vi "pH电极校准.vi"() -> ()   [LabVIEW 2016, in "斯坦道多参数.lvlib"]
uses:
  <vilib>/Utility/miscctls.llb/LVPointTypeDef.ctl
  <vilib>/Analysis/NI_AALBase.lvlib
panel:
  in  "三点标液3":u16(ring)=6 caption="标液3" items=["TECH4.00", "TECH7.00", "TECH10.00", "NIST1.68", "NIST4.01", "NIST6.86", "NIST9.18", "NIST12.68"]
  in  "三点标液2":u16(ring)=5 caption="标液2" items=["TECH4.00", "TECH7.00", "TECH10.00", "NIST1.68", "NIST4.01", "NIST6.86", "NIST9.18", "NIST12.68"]
  in  "三点标液1":u16(ring)=4 caption="标液1" items=["TECH4.00", "TECH7.00", "TECH10.00", "NIST1.68", "NIST4.01", "NIST6.86", "NIST9.18", "NIST12.68"]
  out "第三点校准值":dbl
  in  "校准停止":bool
  in  "校准启动":bool
  out "第二点校准值":dbl
  out "第一点校准值":dbl
  out "提示":string
  in  "校准模式":enum16{"两点校准", "单点校准", "三点校准"}(ring)
  out "最小值":sgl format="%#.2f"
  out "最大值":sgl format="%#.2f"
  out "变异系数":dbl format="%#.6f"
  out "standard deviation":dbl caption="标准差" format="%#.2f"
  out "mean":dbl caption="均值" format="%#.2f"
  out "波形图表":sgl(graph) caption="历史曲线"
  out "当前检测值":dbl format="%#.2g"
  out "标液2":dbl
  out "标液1":dbl
  out "当前信号值":dbl format="%#.2g"
  out "偏移值补偿":dbl format="%#.2g"
  out "电极斜率":dbl
  out "电极零点":dbl
  # "酸碱度电极设定"
  # "mV"
  # "mV"
  # "%"
  # "pH"
  # "请选择校准模式:"
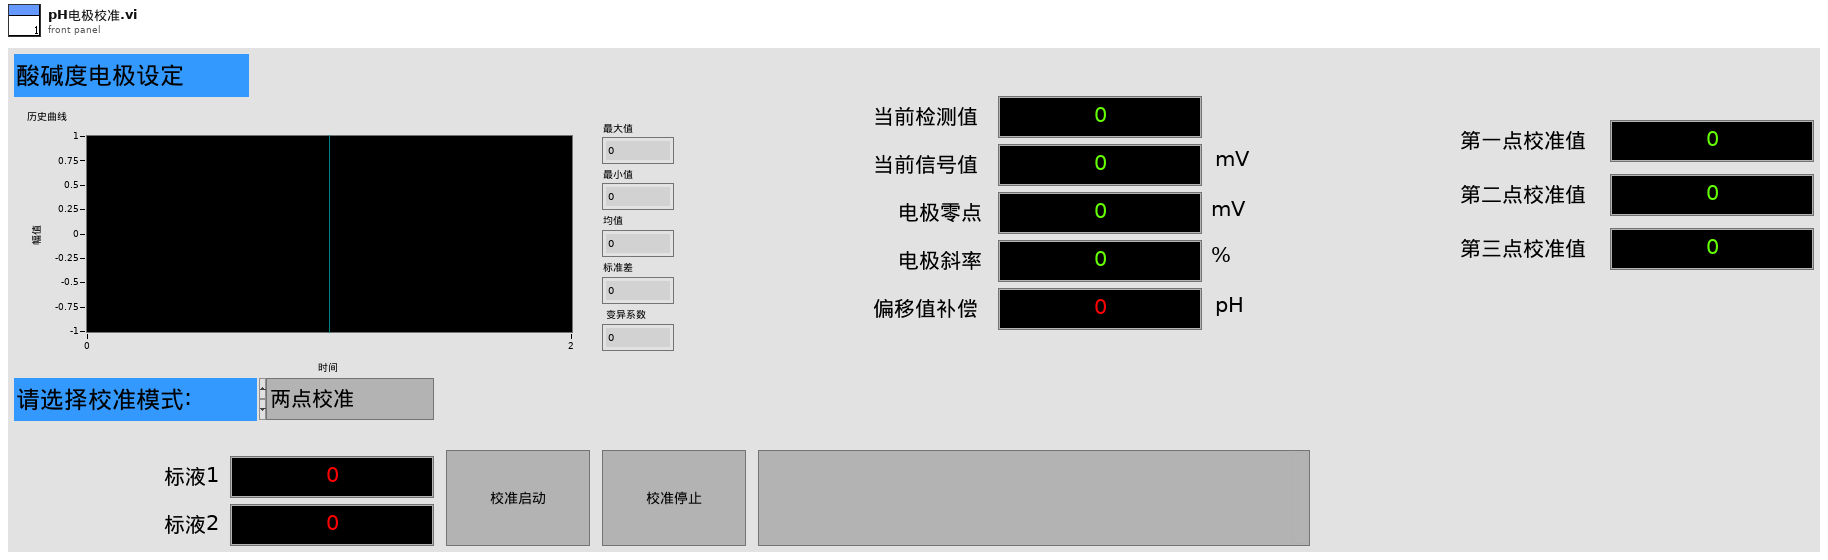
[diagram p1: front panel]
types:
  T1 = typedef "LVPointTypeDef.ctl" = cluster{"Horizontal":i16, "Vertical":i16}
  T2 = typedef "斯坦道多参数.lvlib/校准步骤.ctl" = enum16{"待机", "放置第一点标液", "第一点校准启动", "第一点校准写入", "第一点校准失败", "放置第二点标液", "第二点校准启动", "第二点校准写入", "第二点校准失败", "放置第三点标液", "第三点校准启动", "第三点校准写入", "第三点校准失败", "校准结果写入", "校准结束"}
  T3 = cluster{"电极状态标志":u16, "电极型号标志":u16, "酸碱度测量值":sgl, "温度测量值":sgl, "酸碱度信号值":sgl, "温度信号值":sgl, "酸碱度偏移修正值":sgl, "温度偏移修正值":sgl, "手动温度补偿值":sgl, "酸碱度电极零点":sgl, "酸碱度电极斜率":sgl, "第1点标准值记录":sgl, "第1点信号值记录":sgl, "第1点温度值记录":sgl, "第2点标准值记录":sgl, "第2点信号值记录":sgl, "第2点温度值记录":sgl, "命令滤波设定":u16, "温度模式":enum16{"ATC", "MTC"}, "生产批次":u16, "电极序号":u16, "串口地址":u16, "串口波特率":enum16{"9600", "19200", "115200"}, "串口校验位":enum16{"NONE", "ODD", "EVEN"}, "串口停止位":enum16{"1bit", "2bit"}, "第一点标准值":sgl, "第二点标准值":sgl}
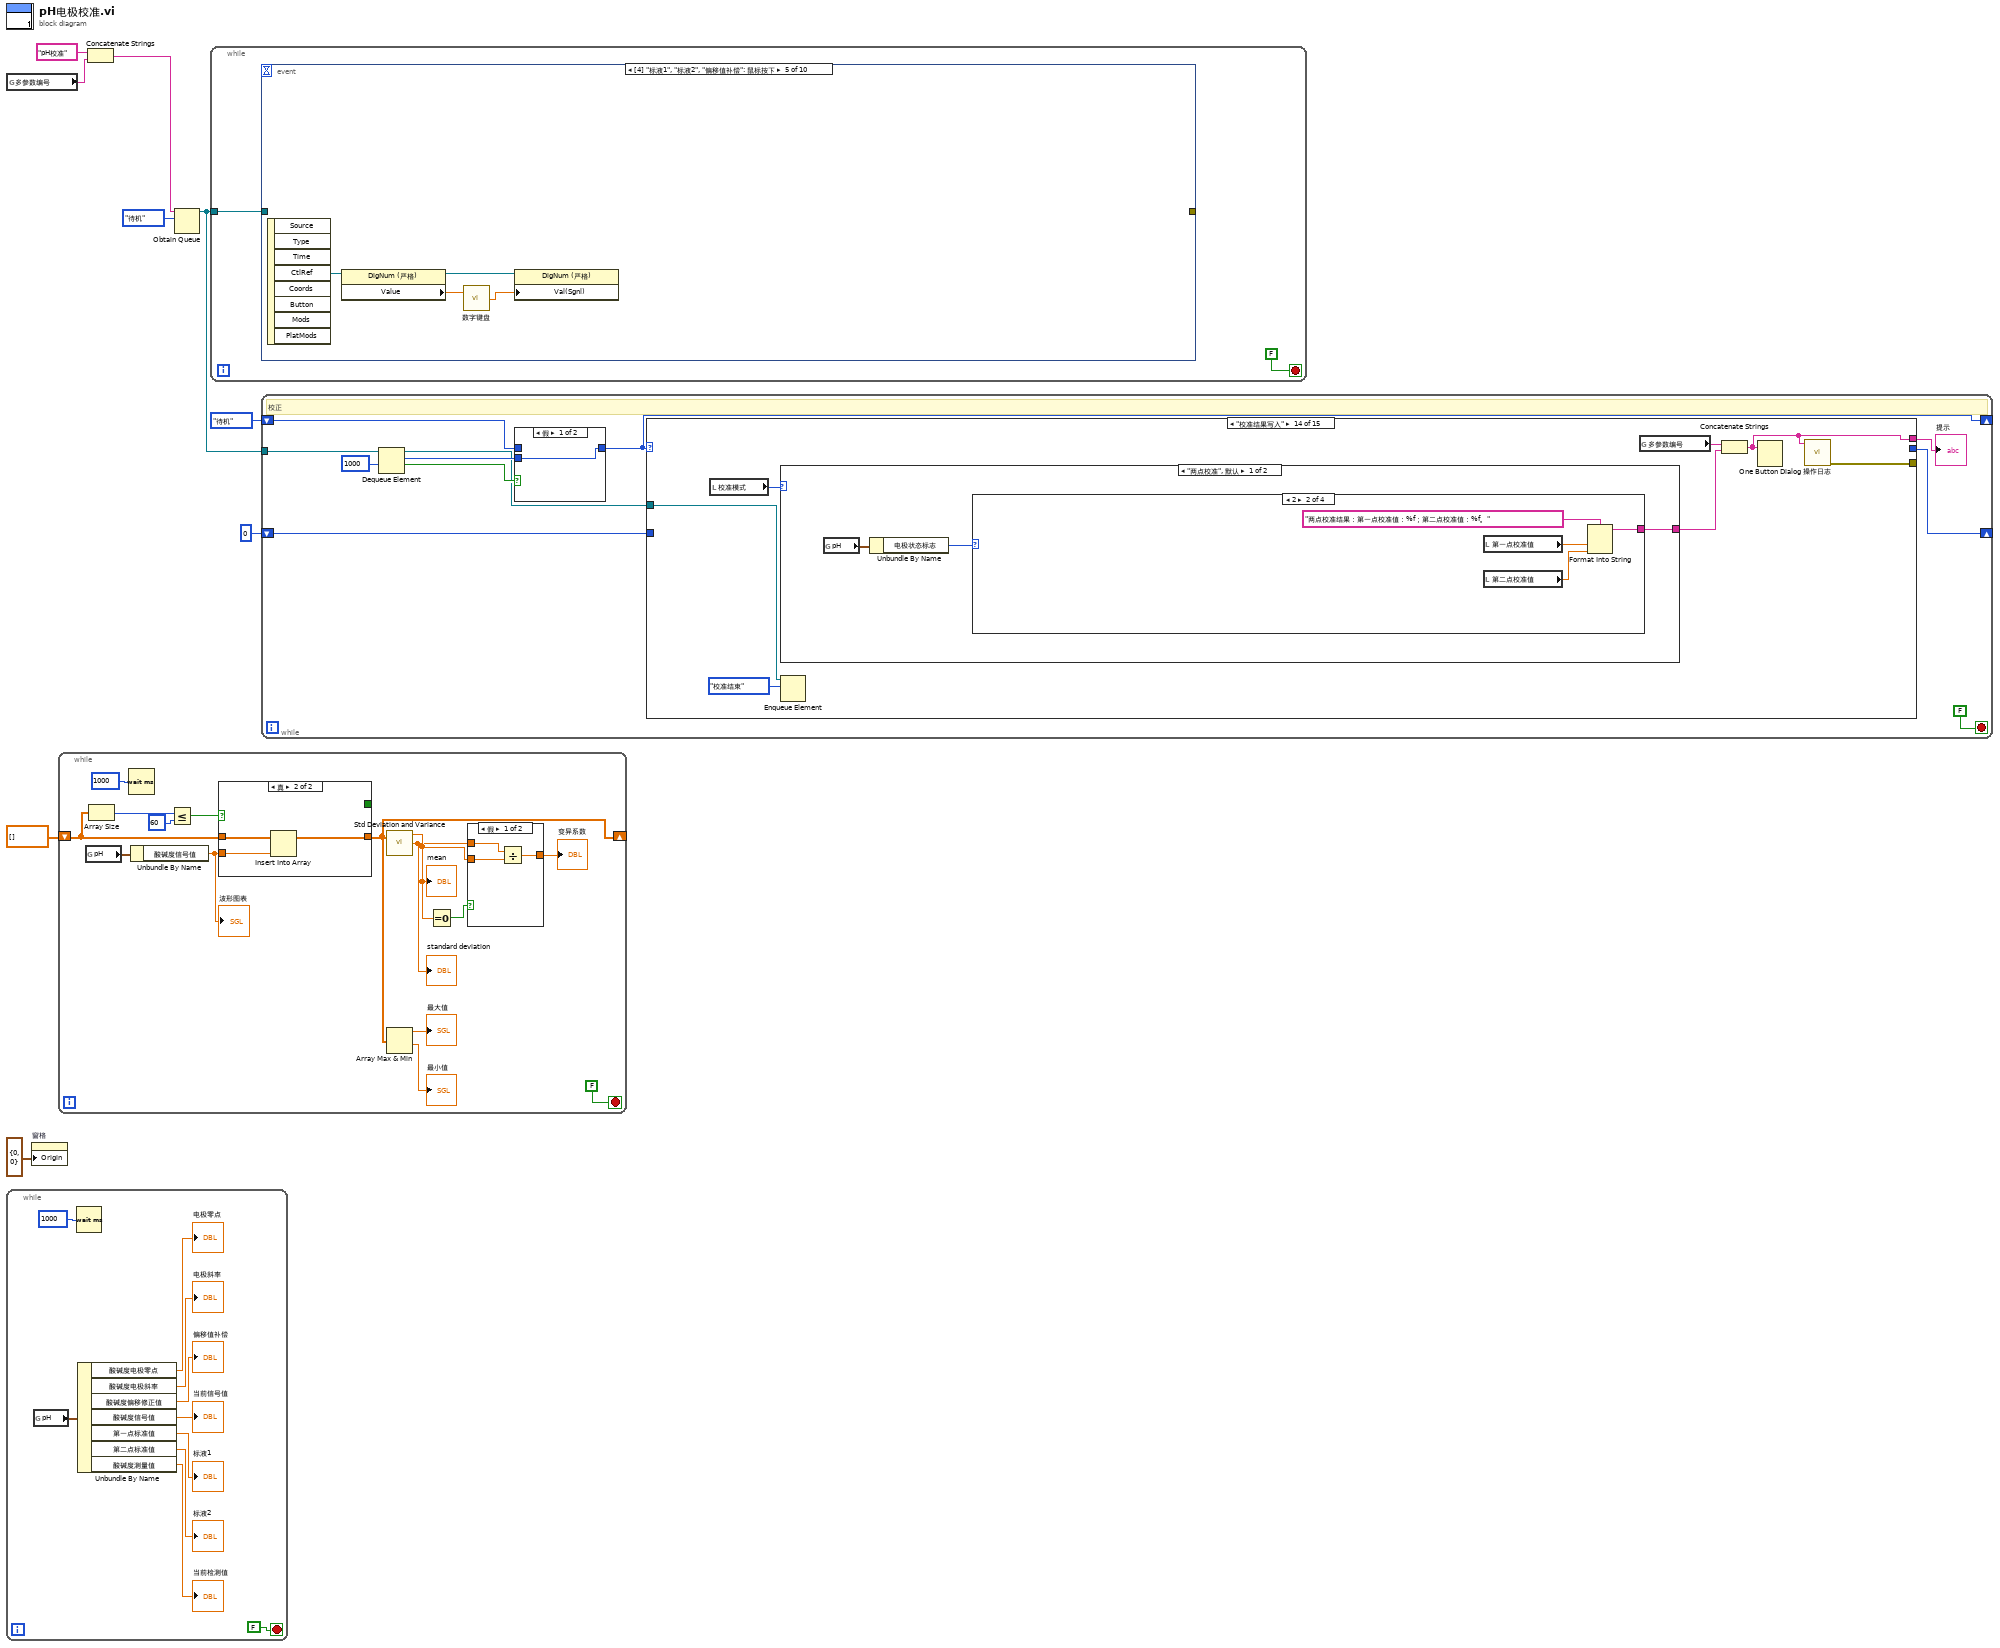
[diagram p0: block diagram]
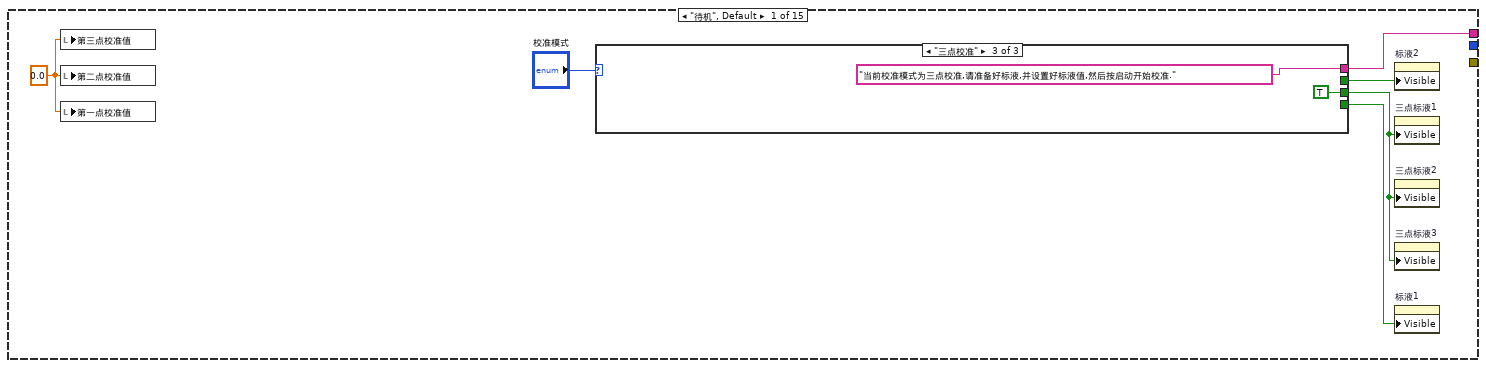
[diagram p3: hidden frame]
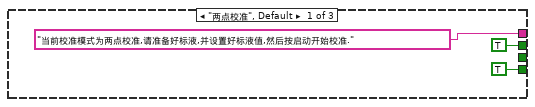
[diagram p4: hidden frame]
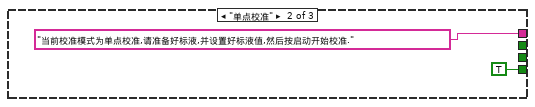
[diagram p5: hidden frame]
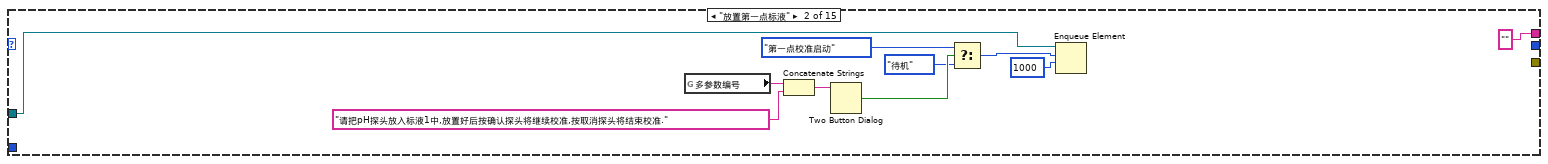
[diagram p6: hidden frame]
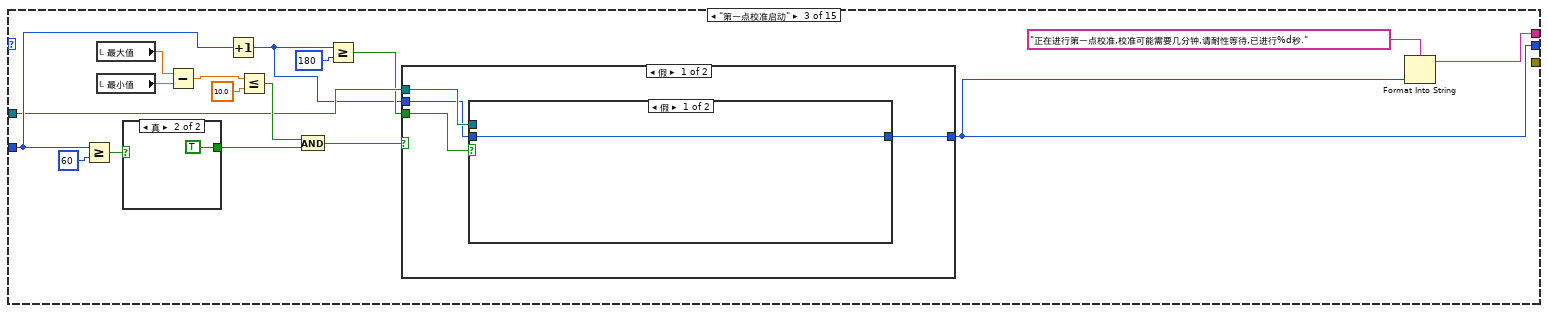
[diagram p7: hidden frame]
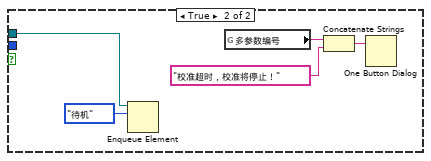
[diagram p8: hidden frame]
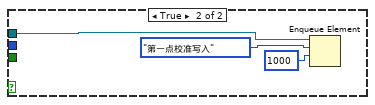
[diagram p9: hidden frame]
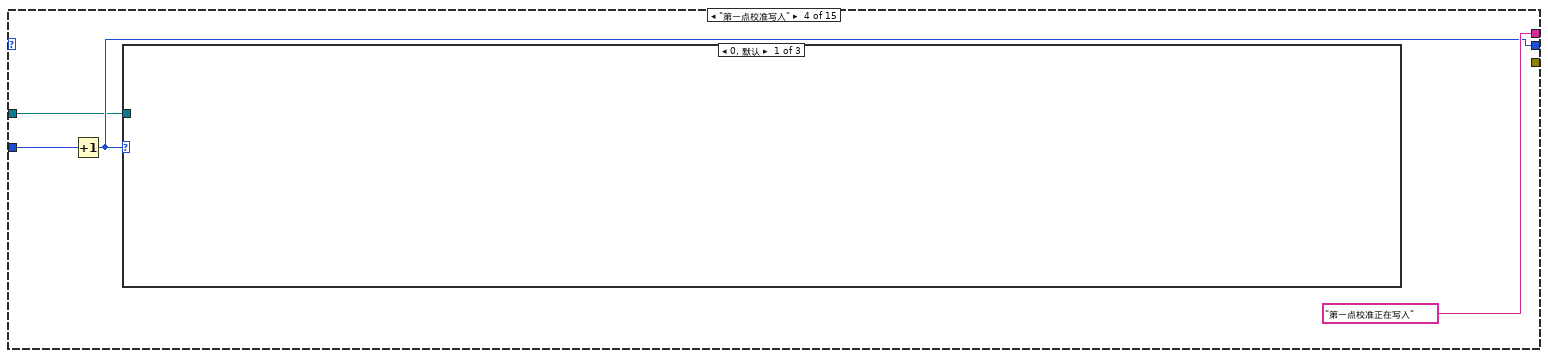
[diagram p11: hidden frame]
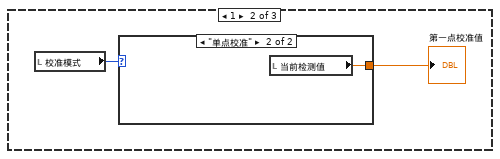
[diagram p12: hidden frame]
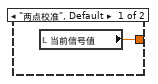
[diagram p13: hidden frame]
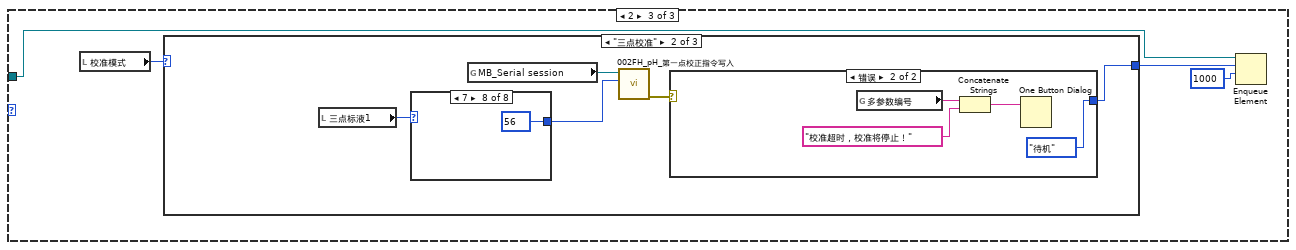
[diagram p14: hidden frame]
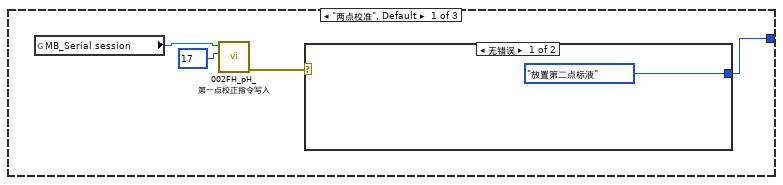
[diagram p15: hidden frame]
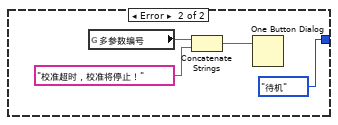
[diagram p16: hidden frame]
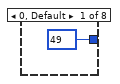
[diagram p17: hidden frame]
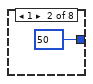
[diagram p18: hidden frame]
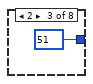
[diagram p19: hidden frame]
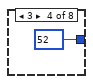
[diagram p20: hidden frame]
diagram:
  n1 = global read "多参数全局变量.vi" "多参数编号"() -> (w1:string)
  n2 = while {
    stop <- FALSE stop-if-true
    n3 = global read "国弘过程全局变量.vi" "pH"() -> (w17:T3)
    n4 = Wait (ms)(milliseconds to wait=u32 1000 ("等待时间（毫秒）")) -> ()  [unwired: 1 out]
    n5 = Unbundle By Name(w17) -> ("酸碱度电极零点"=→"电极零点":sgl, "酸碱度电极斜率"=→"电极斜率":sgl, "酸碱度偏移修正值"=→"偏移值补偿":sgl, "酸碱度信号值"=→"当前信号值":sgl, "第一点标准值"=→"标液1":sgl, "第二点标准值"=→"标液2":sgl, "酸碱度测量值"=→"当前检测值":sgl)
  }
  n6 = property on="窗格" class="Pane"("Origin"=T1 {"Horizontal"=0, "Vertical"=0} ("原点")) -> ()  [unwired: 2 in, 2 out]
  n7 = while {
    shift-right: [w26] -> _
    shift-left: sgl[] [] -> [w30]
    stop <- FALSE stop-if-true
    n8 = global read "国弘过程全局变量.vi" "pH"() -> (w27:T3)
    n9 = Array Size(array=w30) -> (size(s)=w32:i32)
    n10 = Wait (ms)(milliseconds to wait=u32 1000 ("等待时间（毫秒）")) -> ()  [unwired: 1 out]
    n11 = Unbundle By Name(w27) -> ("酸碱度信号值"=w20:sgl)
    "波形图表" <- w20
    n12 = Less Or Equal?(x=w32, y=60) -> (x <= y?=w31:bool)
    n13 = case shown="真" w31 {
      tunnel: w30 -> [w43 w46]
      tunnel: w20 -> [w41 w45]
      tunnel: [w39 w44] -> w26
      tunnel: [TRUE _] -> _
      frame False {
        n14 = Replace Array Subset(array=w43, new element=w41) -> (w42:sgl[])  [unwired: 1 in]
        n15 = Rotate 1D Array(1:w42, 2:-1 ("n")) -> (0:w39:sgl[])
      }
      frame True {
        n16 = Insert Into Array(array=w46, new element=w45) -> (w44:sgl[])  [unwired: 1 in]
      }
    }
    n17 = call <vilib>:"Std Deviation and Variance.vi"("X"=w26) -> ("mean"=w22:dbl, "standard deviation"=w21:dbl)  [unwired: 1 in, 1 out]
    "mean" <- w22
    "standard deviation" <- w21
    n18 = Array Max & Min(array=w26) -> (max value=→"最大值":sgl, min value=→"最小值":sgl)  [unwired: 2 out]
    n19 = Equal To 0?(x=w22) -> (x = 0?=w29:bool)
    n20 = case shown="假" w29 {
      tunnel: w21 -> [w37 _]
      tunnel: [w36 _] -> w23
      tunnel: w22 -> [w35 _]
      frame False {
        n21 = Divide(x=w37, y=w35) -> (x/y=w36:dbl)
      }
      frame True {
      }
    }
    "变异系数" <- w23
  }
  n22 = Concatenate Strings("pH校准" ("名称（未命名）"), w1) -> (w2:string)
  n23 = Obtain Queue(name (unnamed)=w2, element data type=校准步骤."待机" ("枚举")) -> (queue out=w4:refnum<queue>)  [unwired: 3 in, 2 out]
  n24 = while {
    tunnel: w4 -> [w47]
    stop <- FALSE stop-if-true
    n25 = event shown="[4] \"标液1\", \"标液2\", \"偏移值补偿\": 鼠标按下" {
      selector: _ -> [_ _ _ _ _ _ _ _ _ _]
      dyn-events: _ -> [_ _ _ _ _ _ _ _ _ _]
      timeout: _ -> [_ _ _ _ _ _ _ _ _ _]
      tunnel: [_ _ _ _ _ w99 w102 w105 _ _] -> _
      tunnel: w47 -> [_ _ _ _ _ _ _ _ w107 w109]
      event Timeout {
        n26 = event-data() -> ()  [unwired: 1 in, 3 out]
      }
      event "三点标液1": Value Change {
        n27 = event-data() -> ("NewVal"=w49:u16)  [unwired: 1 in, 5 out]
        n28 = case shown="0, 默认" w49 {
          frame 0, Default {
            w50 = u16 0 items=["TECH4.00", "TECH7.00", "TECH10.00", "NIST1.68", "NIST4.01", "NIST6.86", "NIST9.18", "NIST12.68"] ("标液2")
            w51 = u16 2 items=["TECH4.00", "TECH7.00", "TECH10.00", "NIST1.68", "NIST4.01", "NIST6.86", "NIST9.18", "NIST12.68"] ("标液3")
            w52 = u16 1 items=["TECH4.00", "TECH7.00", "TECH10.00", "NIST1.68", "NIST4.01", "NIST6.86", "NIST9.18", "NIST12.68"] ("标液2")
            n29 = local write "三点标液1"(w50) -> ()
            n30 = local write "三点标液2"(w52) -> ()
            n31 = local write "三点标液3"(w51) -> ()
          }
          frame 1 {
            w53 = u16 0 items=["TECH4.00", "TECH7.00", "TECH10.00", "NIST1.68", "NIST4.01", "NIST6.86", "NIST9.18", "NIST12.68"] ("标液2")
            w54 = u16 2 items=["TECH4.00", "TECH7.00", "TECH10.00", "NIST1.68", "NIST4.01", "NIST6.86", "NIST9.18", "NIST12.68"] ("标液3")
            w55 = u16 1 items=["TECH4.00", "TECH7.00", "TECH10.00", "NIST1.68", "NIST4.01", "NIST6.86", "NIST9.18", "NIST12.68"] ("标液2")
            n32 = local write "三点标液1"(w53) -> ()
            n33 = local write "三点标液2"(w55) -> ()
            n34 = local write "三点标液3"(w54) -> ()
          }
          frame 2 {
            w56 = u16 2 items=["TECH4.00", "TECH7.00", "TECH10.00", "NIST1.68", "NIST4.01", "NIST6.86", "NIST9.18", "NIST12.68"] ("标液2")
            w57 = u16 0 items=["TECH4.00", "TECH7.00", "TECH10.00", "NIST1.68", "NIST4.01", "NIST6.86", "NIST9.18", "NIST12.68"] ("标液3")
            w58 = u16 1 items=["TECH4.00", "TECH7.00", "TECH10.00", "NIST1.68", "NIST4.01", "NIST6.86", "NIST9.18", "NIST12.68"] ("标液2")
            n35 = local write "三点标液1"(w56) -> ()
            n36 = local write "三点标液2"(w58) -> ()
            n37 = local write "三点标液3"(w57) -> ()
          }
          frame 3 {
            w59 = u16 3 items=["TECH4.00", "TECH7.00", "TECH10.00", "NIST1.68", "NIST4.01", "NIST6.86", "NIST9.18", "NIST12.68"] ("标液2")
            w60 = u16 5 items=["TECH4.00", "TECH7.00", "TECH10.00", "NIST1.68", "NIST4.01", "NIST6.86", "NIST9.18", "NIST12.68"] ("标液3")
            w61 = u16 4 items=["TECH4.00", "TECH7.00", "TECH10.00", "NIST1.68", "NIST4.01", "NIST6.86", "NIST9.18", "NIST12.68"] ("标液2")
            n38 = local write "三点标液1"(w59) -> ()
            n39 = local write "三点标液2"(w61) -> ()
            n40 = local write "三点标液3"(w60) -> ()
          }
          frame 4 {
            w62 = u16 4 items=["TECH4.00", "TECH7.00", "TECH10.00", "NIST1.68", "NIST4.01", "NIST6.86", "NIST9.18", "NIST12.68"] ("标液2")
            w63 = u16 6 items=["TECH4.00", "TECH7.00", "TECH10.00", "NIST1.68", "NIST4.01", "NIST6.86", "NIST9.18", "NIST12.68"] ("标液3")
            w64 = u16 5 items=["TECH4.00", "TECH7.00", "TECH10.00", "NIST1.68", "NIST4.01", "NIST6.86", "NIST9.18", "NIST12.68"] ("标液2")
            n41 = local write "三点标液1"(w62) -> ()
            n42 = local write "三点标液2"(w64) -> ()
            n43 = local write "三点标液3"(w63) -> ()
          }
          frame 5..7 {
            w65 = u16 5 items=["TECH4.00", "TECH7.00", "TECH10.00", "NIST1.68", "NIST4.01", "NIST6.86", "NIST9.18", "NIST12.68"] ("标液2")
            w66 = u16 7 items=["TECH4.00", "TECH7.00", "TECH10.00", "NIST1.68", "NIST4.01", "NIST6.86", "NIST9.18", "NIST12.68"] ("标液3")
            w67 = u16 6 items=["TECH4.00", "TECH7.00", "TECH10.00", "NIST1.68", "NIST4.01", "NIST6.86", "NIST9.18", "NIST12.68"] ("标液2")
            n44 = local write "三点标液1"(w65) -> ()
            n45 = local write "三点标液2"(w67) -> ()
            n46 = local write "三点标液3"(w66) -> ()
          }
        }
      }
      event "三点标液2": Value Change {
        n47 = event-data() -> ("NewVal"=w68:u16)  [unwired: 1 in, 5 out]
        n48 = case shown="6, 7" w68 {
          frame 0..2, Default {
            w69 = u16 0 items=["TECH4.00", "TECH7.00", "TECH10.00", "NIST1.68", "NIST4.01", "NIST6.86", "NIST9.18", "NIST12.68"] ("标液2")
            w70 = u16 2 items=["TECH4.00", "TECH7.00", "TECH10.00", "NIST1.68", "NIST4.01", "NIST6.86", "NIST9.18", "NIST12.68"] ("标液3")
            w71 = u16 1 items=["TECH4.00", "TECH7.00", "TECH10.00", "NIST1.68", "NIST4.01", "NIST6.86", "NIST9.18", "NIST12.68"] ("标液2")
            n49 = local write "三点标液1"(w69) -> ()
            n50 = local write "三点标液2"(w71) -> ()
            n51 = local write "三点标液3"(w70) -> ()
          }
          frame 3, 4 {
            w72 = u16 3 items=["TECH4.00", "TECH7.00", "TECH10.00", "NIST1.68", "NIST4.01", "NIST6.86", "NIST9.18", "NIST12.68"] ("标液2")
            w73 = u16 5 items=["TECH4.00", "TECH7.00", "TECH10.00", "NIST1.68", "NIST4.01", "NIST6.86", "NIST9.18", "NIST12.68"] ("标液3")
            w74 = u16 4 items=["TECH4.00", "TECH7.00", "TECH10.00", "NIST1.68", "NIST4.01", "NIST6.86", "NIST9.18", "NIST12.68"] ("标液2")
            n52 = local write "三点标液1"(w72) -> ()
            n53 = local write "三点标液2"(w74) -> ()
            n54 = local write "三点标液3"(w73) -> ()
          }
          frame 5 {
            w75 = u16 6 items=["TECH4.00", "TECH7.00", "TECH10.00", "NIST1.68", "NIST4.01", "NIST6.86", "NIST9.18", "NIST12.68"] ("标液3")
            w76 = u16 5 items=["TECH4.00", "TECH7.00", "TECH10.00", "NIST1.68", "NIST4.01", "NIST6.86", "NIST9.18", "NIST12.68"] ("标液2")
            n55 = local write "三点标液2"(w76) -> ()
            n56 = local write "三点标液3"(w75) -> ()
          }
          frame 6, 7 {
            w77 = u16 7 items=["TECH4.00", "TECH7.00", "TECH10.00", "NIST1.68", "NIST4.01", "NIST6.86", "NIST9.18", "NIST12.68"] ("标液3")
            w78 = u16 6 items=["TECH4.00", "TECH7.00", "TECH10.00", "NIST1.68", "NIST4.01", "NIST6.86", "NIST9.18", "NIST12.68"] ("标液2")
            n57 = local write "三点标液2"(w78) -> ()
            n58 = local write "三点标液3"(w77) -> ()
          }
        }
      }
      event "三点标液3": Value Change {
        n59 = event-data() -> ("NewVal"=w79:u16)  [unwired: 1 in, 5 out]
        n60 = case shown="3..7" w79 {
          frame 0, 1, Default {
            w80 = u16 2 items=["TECH4.00", "TECH7.00", "TECH10.00", "NIST1.68", "NIST4.01", "NIST6.86", "NIST9.18", "NIST12.68"] ("标液2")
            w81 = u16 0 items=["TECH4.00", "TECH7.00", "TECH10.00", "NIST1.68", "NIST4.01", "NIST6.86", "NIST9.18", "NIST12.68"] ("标液3")
            w82 = u16 1 items=["TECH4.00", "TECH7.00", "TECH10.00", "NIST1.68", "NIST4.01", "NIST6.86", "NIST9.18", "NIST12.68"] ("标液2")
            n61 = local write "三点标液1"(w80) -> ()
            n62 = local write "三点标液2"(w82) -> ()
            n63 = local write "三点标液3"(w81) -> ()
          }
          frame 2 {
            w83 = u16 0 items=["TECH4.00", "TECH7.00", "TECH10.00", "NIST1.68", "NIST4.01", "NIST6.86", "NIST9.18", "NIST12.68"] ("标液2")
            w84 = u16 2 items=["TECH4.00", "TECH7.00", "TECH10.00", "NIST1.68", "NIST4.01", "NIST6.86", "NIST9.18", "NIST12.68"] ("标液3")
            w85 = u16 1 items=["TECH4.00", "TECH7.00", "TECH10.00", "NIST1.68", "NIST4.01", "NIST6.86", "NIST9.18", "NIST12.68"] ("标液2")
            n64 = local write "三点标液1"(w83) -> ()
            n65 = local write "三点标液2"(w85) -> ()
            n66 = local write "三点标液3"(w84) -> ()
          }
          frame 3..7 {
            n67 = local read "三点标液1"() -> (w88:u16)
            n68 = local read "三点标液2"() -> (w87:u16)
            n69 = Less?(x=w88, y=w87) -> (x < y?=w86:bool)
            n70 = case shown="假" w86 {
              frame False {
              }
              frame True {
                n71 = local read "三点标液3"() -> (w91:u16)
                n72 = local read "三点标液2"() -> (w89:u16)
                n73 = Less Or Equal?(x=w91, y=w89) -> (x <= y?=w90:bool)
                n74 = case shown="真" w90 {
                  tunnel: w89 -> [_ w93]
                  frame False {
                  }
                  frame True {
                    n75 = Increment(x=w93) -> (x+1=w92:u16)
                    n76 = local write "三点标液3"(w92) -> ()
                  }
                }
              }
            }
          }
        }
      }
      event "标液1", "标液2", "偏移值补偿": Mouse Down {
        n77 = event-data() -> ("CtlRef"=w97:refnum<vi>)  [unwired: 1 in, 7 out]
        n78 = property class="DigNum (严格)"(reference=w97) -> (reference out=w94:refnum<vi>, "Value"=w95:dbl)  [unwired: 1 in, 1 out]
        n79 = call "数字键盘.vi"("OldNumber"=w95) -> ("NewNumber"=w96:dbl)  [unwired: 1 in]
        n80 = property class="DigNum (严格)"(reference=w94, "Val(Sgnl)"=w96) -> ()  [unwired: 1 in, 2 out]
      }
      event "偏移值补偿": Value Change {
        n81 = event-data() -> ("NewVal"=w100:dbl)  [unwired: 1 in, 5 out]
        n82 = global read "多参数全局变量.vi" "MB_Serial session"() -> (w98:refnum<class "MB_Master_Serial.lvclass">)
        n83 = call "000CH_pH_pH偏移修正值写入.vi"("数值"=w100, "MB_Serial session in"=w98) -> ("error out"=w99:errorcluster)  [unwired: 8 in, 1 out]
      }
      event "标液1": Value Change {
        n84 = event-data() -> ("NewVal"=w103:dbl)  [unwired: 1 in, 5 out]
        n85 = global read "多参数全局变量.vi" "MB_Serial session"() -> (w101:refnum<class "MB_Master_Serial.lvclass">)
        n86 = call "0030H_pH_第一点标准值写入.vi"("数值"=w103, "MB_Serial session in"=w101) -> ("error out"=w102:errorcluster)  [unwired: 8 in, 1 out]
      }
      event "标液2": Value Change {
        n87 = event-data() -> ("NewVal"=w106:dbl)  [unwired: 1 in, 5 out]
        n88 = global read "多参数全局变量.vi" "MB_Serial session"() -> (w104:refnum<class "MB_Master_Serial.lvclass">)
        n89 = call "0033H_pH_第二点标准值写入.vi"("数值"=w106, "MB_Serial session in"=w104) -> ("error out"=w105:errorcluster)  [unwired: 8 in, 1 out]
      }
      event "校准启动": Value Change {
        n90 = event-data() -> ()  [unwired: 1 in, 6 out]
        n91 = Enqueue Element(queue=w107, element=校准步骤."放置第一点标液" ("元素")) -> ()  [unwired: 2 in, 3 out]
      }
      event "校准停止": Value Change {
        n92 = event-data() -> ()  [unwired: 1 in, 6 out]
        n93 = Flush Queue(queue=w109) -> (queue out=w110:refnum<queue>)  [unwired: 1 in, 2 out]
        n94 = Enqueue Element(queue=w110, element=校准步骤."待机" ("元素"), timeout in ms (-1)=1000 ("超时毫秒(-1)")) -> ()  [unwired: 1 in, 3 out]
      }
    }
  }
  n95 = while "While循环" {
    shift-right: [w114] -> _
    shift-left: 校准步骤."待机" ("枚举") -> [w115]
    shift-right: [w121] -> _
    shift-left: 0 -> [w122]
    tunnel: w4 -> [w119]
    stop <- FALSE stop-if-true
    # "校正"
    n96 = Dequeue Element(queue=w119, timeout in ms (-1)=1000 ("超时毫秒(-1)")) -> (queue out=w113:refnum<queue>, element=w116:T2, timed out?=w117:bool)  [unwired: 1 in, 1 out]
    n97 = case shown="假" w117 {
      tunnel: w116 -> [w124 _]
      tunnel: [w124 w125] -> w114
      tunnel: w115 -> [_ w125]
      frame False {
      }
      frame True {
      }
    }
    n98 = case shown="\"校准结果写入\"" w114 {
      tunnel: [w131 "" ("提示") w164 "第一点校准正在写入" ("提示") _ "" ("提示") w245 "第二点校准正在写入" ("提示") _ "" ("提示") w322 "第三点校准正在写入" ("提示") _ w363 w402] -> w120
      tunnel: w122 -> [_ _ w158 w182 _ _ w239 w263 _ _ w316 w340 _ _ _]
      tunnel: [_ _ w149 w181 _ _ w230 w262 _ _ w307 w339 _ _ _] -> w121
      tunnel: w113 -> [_ w148 w152 w180 _ w229 w233 w261 _ w306 w310 w338 _ w369 _]
      tunnel: [_ _ _ _ _ _ _ _ _ _ _ _ _ w365 _] -> _
      frame "待机", Default {
        w127 = 0.0 ("第一点校准值")
        n99 = local write "第三点校准值"(w127) -> ()
        n100 = local write "第二点校准值"(w127) -> ()
        n101 = local write "第一点校准值"(w127) -> ()
        n102 = case shown="\"三点校准\"" "校准模式" {
          tunnel: ["当前校准模式为两点校准,请准备好标液,并设置好标液值,然后按启动开始校准." ("提示") "当前校准模式为单点校准,请准备好标液,并设置好标液值,然后按启动开始校准." ("提示") "当前校准模式为三点校准,请准备好标液,并设置好标液值,然后按启动开始校准." ("提示")] -> w131
          tunnel: [TRUE ("可见") _ _] -> w130
          tunnel: [TRUE ("可见") TRUE ("可见") _] -> w128
          tunnel: [_ _ TRUE ("可见")] -> w126
          frame "两点校准", Default {
          }
          frame "单点校准" {
          }
          frame "三点校准" {
          }
        }
        n103 = property on="标液2" class="DigNum (严格)"("Visible"=w130) -> ()  [unwired: 2 in, 2 out]
        n104 = property on="三点标液1" class="Ring (严格)"("Visible"=w126) -> ()  [unwired: 2 in, 2 out]
        n105 = property on="三点标液2" class="Ring (严格)"("Visible"=w126) -> ()  [unwired: 2 in, 2 out]
        n106 = property on="三点标液3" class="Ring (严格)"("Visible"=w126) -> ()  [unwired: 2 in, 2 out]
        n107 = property on="标液1" class="DigNum (严格)"("Visible"=w128) -> ()  [unwired: 2 in, 2 out]
      }
      frame "放置第一点标液" {
        n108 = global read "多参数全局变量.vi" "多参数编号"() -> (w139:string)
        n109 = Concatenate Strings(w139, "请把pH探头放入标液1中,放置好后按确认探头将继续校准,按取消探头将结束校准." ("消息")) -> (w140:string)
        n110 = Two Button Dialog(message=w140) -> (T button?=w146:bool)  [unwired: 2 in]
        n111 = Select(t=校准步骤."第一点校准启动" ("元素"), s=w146, f=校准步骤."待机" ("元素")) -> (s? t:f=w143:T2)
        n112 = Enqueue Element(queue=w148, element=w143, timeout in ms (-1)=1000 ("超时毫秒(-1)")) -> ()  [unwired: 1 in, 3 out]
      }
      frame "第一点校准启动" {
        n113 = Greater Or Equal?(x=w158, y=60) -> (x >= y?=w159:bool)
        n114 = local read "最大值"() -> (w155:sgl)
        n115 = local read "最小值"() -> (w156:sgl)
        n116 = case shown="真" w159 {
          tunnel: [_ TRUE] -> w157
          frame False {
          }
          frame True {
          }
        }
        n117 = Subtract(x=w155, y=w156) -> (x-y=w154:sgl)
        n118 = Increment(x=w158) -> (x+1=w150:i32)
        n119 = Less Or Equal?(x=w154, y=10.0) -> (x <= y?=w162:bool)
        n120 = And(x=w162, y=w157) -> (x .and. y?=w153:bool)
        n121 = Greater Or Equal?(x=w150, y=180) -> (x >= y?=w151:bool)
        n122 = case shown="假" w153 {
          tunnel: w152 -> [w168 w178]
          tunnel: w151 -> [w169 _]
          tunnel: w150 -> [w167 _]
          tunnel: [w166 _] -> w149
          frame False {
            n123 = case shown="假" w169 {
              tunnel: w168 -> [_ w175]
              tunnel: w167 -> [w170 _]
              tunnel: [w170 _] -> w166
              frame False {
              }
              frame True {
                n124 = Enqueue Element(queue=w175, element=校准步骤."待机" ("元素")) -> ()  [unwired: 2 in, 3 out]
                n125 = global read "多参数全局变量.vi" "多参数编号"() -> (w171:string)
                n126 = Concatenate Strings(w171, "校准超时，校准将停止！" ("消息")) -> (w172:string)
                n127 = One Button Dialog(message=w172) -> ()  [unwired: 1 in, 1 out]
              }
            }
          }
          frame True {
            n128 = Enqueue Element(queue=w178, element=校准步骤."第一点校准写入" ("元素"), timeout in ms (-1)=1000 ("超时毫秒(-1)")) -> ()  [unwired: 1 in, 3 out]
          }
        }
        n129 = Format Into String(format string="正在进行第一点校准,校准可能需要几分钟,请耐性等待,已进行%d秒." ("格式字符串"), w149) -> (resulting string=w164:string)  [unwired: 2 in, 1 out]
      }
      frame "第一点校准写入" {
        n130 = Increment(x=w182) -> (x+1=w181:i32)
        n131 = case shown="0, 默认" w181 {
          tunnel: w180 -> [_ _ w191]
          frame 0, Default {
          }
          frame 1 {
            n132 = local read "校准模式"() -> (w184:enum16{"两点校准", "单点校准", "三点校准"})
            n133 = case shown="\"单点校准\"" w184 {
              tunnel: [w186 w187] -> w185
              frame "两点校准", Default {
                n134 = local read "当前信号值"() -> (w186:dbl)
              }
              frame "单点校准" {
                n135 = local read "当前检测值"() -> (w187:dbl)
              }
            }
            "第一点校准值" <- w185
          }
          frame 2 {
            n136 = local read "校准模式"() -> (w190:enum16{"两点校准", "单点校准", "三点校准"})
            n137 = case shown="\"三点校准\"" w190 {
              tunnel: [w195 w205 校准步骤."校准结果写入" ("元素")] -> w189
              frame "两点校准", Default {
                n138 = global read "多参数全局变量.vi" "MB_Serial session"() -> (w194:refnum<class "MB_Master_Serial.lvclass">)
                n139 = call "002FH_pH_第一点校正指令写入.vi"("数值"=u16 17, "MB_Serial session in"=w194) -> ("error out"=w192:errorcluster)  [unwired: 8 in, 1 out]
                n140 = case shown="无错误" w192 {
                  tunnel: [校准步骤."放置第二点标液" ("元素") 校准步骤."待机" ("元素")] -> w195
                  frame No Error {
                  }
                  frame Error {
                    n141 = global read "多参数全局变量.vi" "多参数编号"() -> (w197:string)
                    n142 = Concatenate Strings(w197, "校准超时，校准将停止！" ("消息")) -> (w198:string)
                    n143 = One Button Dialog(message=w198) -> ()  [unwired: 1 in, 1 out]
                  }
                }
              }
              frame "三点校准" {
                n144 = local read "三点标液1"() -> (w202:u16)
                n145 = case shown="7" w202 {
                  tunnel: [u16 49 ("数值") u16 50 ("数值") u16 51 ("数值") u16 52 ("数值") u16 53 ("数值") u16 54 ("数值") u16 55 ("数值") u16 56 ("数值")] -> w201
                  frame 0, Default {
                  }
                  frame 1 {
                  }
                  frame 2 {
                  }
                  frame 3 {
                  }
                  frame 4 {
                  }
                  frame 5 {
                  }
                  frame 6 {
                  }
                  frame 7 {
                  }
                }
                n146 = global read "多参数全局变量.vi" "MB_Serial session"() -> (w204:refnum<class "MB_Master_Serial.lvclass">)
                n147 = call "002FH_pH_第一点校正指令写入.vi"("数值"=w201, "MB_Serial session in"=w204) -> ("error out"=w203:errorcluster)  [unwired: 8 in, 1 out]
                n148 = case shown="错误" w203 {
                  tunnel: [校准步骤."放置第二点标液" ("元素") 校准步骤."待机" ("元素")] -> w205
                  frame No Error {
                  }
                  frame Error {
                    n149 = global read "多参数全局变量.vi" "多参数编号"() -> (w215:string)
                    n150 = Concatenate Strings(w215, "校准超时，校准将停止！" ("消息")) -> (w216:string)
                    n151 = One Button Dialog(message=w216) -> ()  [unwired: 1 in, 1 out]
                  }
                }
              }
              frame "单点校准" {
              }
            }
            n152 = Enqueue Element(queue=w191, element=w189, timeout in ms (-1)=1000 ("超时毫秒(-1)")) -> ()  [unwired: 1 in, 3 out]
          }
        }
      }
      frame "第一点校准失败" {
      }
      frame "放置第二点标液" {
        n153 = global read "多参数全局变量.vi" "多参数编号"() -> (w220:string)
        n154 = Concatenate Strings(w220, "请把探头放入标液2中,放置好后按确认探头将继续校准,按取消探头将结束校准." ("消息")) -> (w221:string)
        n155 = Two Button Dialog(message=w221) -> (T button?=w227:bool)  [unwired: 2 in]
        n156 = Select(t=校准步骤."第二点校准启动" ("元素"), s=w227, f=校准步骤."待机" ("元素")) -> (s? t:f=w224:T2)
        n157 = Enqueue Element(queue=w229, element=w224, timeout in ms (-1)=1000 ("超时毫秒(-1)")) -> ()  [unwired: 1 in, 3 out]
      }
      frame "第二点校准启动" {
        n158 = Greater Or Equal?(x=w239, y=60) -> (x >= y?=w240:bool)
        n159 = local read "最大值"() -> (w236:sgl)
        n160 = local read "最小值"() -> (w237:sgl)
        n161 = case shown="真" w240 {
          tunnel: [_ TRUE] -> w238
          frame False {
          }
          frame True {
          }
        }
        n162 = Subtract(x=w236, y=w237) -> (x-y=w235:sgl)
        n163 = Increment(x=w239) -> (x+1=w231:i32)
        n164 = Less Or Equal?(x=w235, y=10.0) -> (x <= y?=w243:bool)
        n165 = And(x=w243, y=w238) -> (x .and. y?=w234:bool)
        n166 = Greater Or Equal?(x=w231, y=180) -> (x >= y?=w232:bool)
        n167 = case shown="假" w234 {
          tunnel: w233 -> [w249 w259]
          tunnel: w232 -> [w250 _]
          tunnel: w231 -> [w248 _]
          tunnel: [w247 _] -> w230
          frame False {
            n168 = case shown="真" w250 {
              tunnel: w249 -> [_ w256]
              tunnel: w248 -> [w251 _]
              tunnel: [w251 _] -> w247
              frame False {
              }
              frame True {
                n169 = global read "多参数全局变量.vi" "多参数编号"() -> (w252:string)
                n170 = Enqueue Element(queue=w256, element=校准步骤."放置第二点标液" ("元素")) -> ()  [unwired: 2 in, 3 out]
                n171 = Concatenate Strings(w252, "校准超时，校准将停止！" ("消息")) -> (w253:string)
                n172 = One Button Dialog(message=w253) -> ()  [unwired: 1 in, 1 out]
              }
            }
          }
          frame True {
            n173 = Enqueue Element(queue=w259, element=校准步骤."第二点校准写入" ("元素"), timeout in ms (-1)=1000 ("超时毫秒(-1)")) -> ()  [unwired: 1 in, 3 out]
          }
        }
        n174 = Format Into String(format string="正在进行第二点校准,校准可能需要几分钟,请耐性等待,已进行%d秒." ("格式字符串"), w230) -> (resulting string=w245:string)  [unwired: 2 in, 1 out]
      }
      frame "第二点校准写入" {
        n175 = Increment(x=w263) -> (x+1=w262:i32)
        n176 = case shown="2" w262 {
          tunnel: w261 -> [_ _ w269]
          frame 0, Default {
          }
          frame 1 {
            n177 = local read "当前信号值"() -> (→"第二点校准值":dbl)
          }
          frame 2 {
            n178 = local read "校准模式"() -> (w266:enum16{"两点校准", "单点校准", "三点校准"})
            n179 = case shown="\"三点校准\"" w266 {
              tunnel: [w270 w281] -> w267
              frame "两点校准", Default {
                n180 = global read "多参数全局变量.vi" "MB_Serial session"() -> (w272:refnum<class "MB_Master_Serial.lvclass">)
                n181 = call "0032H_pH_第二点校正指令写入.vi"("数值"=u16 33, "MB_Serial session in"=w272) -> ("error out"=w271:errorcluster)  [unwired: 8 in, 1 out]
                n182 = case shown="错误" w271 {
                  tunnel: [校准步骤."校准结果写入" ("元素") 校准步骤."放置第二点标液" ("元素")] -> w270
                  frame No Error {
                  }
                  frame Error {
                    n183 = global read "多参数全局变量.vi" "多参数编号"() -> (w277:string)
                    n184 = Format Into String(format string="%s校准超时，校准将停止！" ("消息"), w277) -> (resulting string=w275:string)  [unwired: 2 in, 1 out]
                    n185 = One Button Dialog(message=w275) -> ()  [unwired: 1 in, 1 out]
                  }
                }
              }
              frame "三点校准" {
                n186 = local read "三点标液2"() -> (w280:u16)
                n187 = case shown="7" w280 {
                  tunnel: [u16 49 ("数值") u16 50 ("数值") u16 51 ("数值") u16 52 ("数值") u16 53 ("数值") u16 54 ("数值") u16 55 ("数值") u16 56 ("数值")] -> w279
                  frame 0, Default {
                  }
                  frame 1 {
                  }
                  frame 2 {
                  }
                  frame 3 {
                  }
                  frame 4 {
                  }
                  frame 5 {
                  }
                  frame 6 {
                  }
                  frame 7 {
                  }
                }
                n188 = global read "多参数全局变量.vi" "MB_Serial session"() -> (w283:refnum<class "MB_Master_Serial.lvclass">)
                n189 = call "0032H_pH_第二点校正指令写入.vi"("数值"=w279, "MB_Serial session in"=w283) -> ("error out"=w282:errorcluster)  [unwired: 8 in, 1 out]
                n190 = case shown="错误" w282 {
                  tunnel: [校准步骤."放置第三点标液" ("元素") 校准步骤."待机" ("元素")] -> w281
                  frame No Error {
                  }
                  frame Error {
                    n191 = global read "多参数全局变量.vi" "多参数编号"() -> (w293:string)
                    n192 = Concatenate Strings(w293, "校准超时，校准将停止！" ("消息")) -> (w294:string)
                    n193 = One Button Dialog(message=w294) -> ()  [unwired: 1 in, 1 out]
                  }
                }
              }
            }
            n194 = Enqueue Element(queue=w269, element=w267, timeout in ms (-1)=1000 ("超时毫秒(-1)")) -> ()  [unwired: 1 in, 3 out]
          }
        }
      }
      frame "第二点校准失败" {
      }
      frame "放置第三点标液" {
        n195 = global read "多参数全局变量.vi" "多参数编号"() -> (w297:string)
        n196 = Concatenate Strings(w297, "请把探头放入标液3中,放置好后按确认探头将继续校准,按取消探头将结束校准." ("消息")) -> (w298:string)
        n197 = Two Button Dialog(message=w298) -> (T button?=w304:bool)  [unwired: 2 in]
        n198 = Select(t=校准步骤."第三点校准启动" ("元素"), s=w304, f=校准步骤."待机" ("元素")) -> (s? t:f=w301:T2)
        n199 = Enqueue Element(queue=w306, element=w301, timeout in ms (-1)=1000 ("超时毫秒(-1)")) -> ()  [unwired: 1 in, 3 out]
      }
      frame "第三点校准启动" {
        n200 = Greater Or Equal?(x=w316, y=60) -> (x >= y?=w317:bool)
        n201 = local read "最大值"() -> (w313:sgl)
        n202 = local read "最小值"() -> (w314:sgl)
        n203 = case shown="真" w317 {
          tunnel: [_ TRUE] -> w315
          frame False {
          }
          frame True {
          }
        }
        n204 = Subtract(x=w313, y=w314) -> (x-y=w312:sgl)
        n205 = Increment(x=w316) -> (x+1=w308:i32)
        n206 = Less Or Equal?(x=w312, y=10.0) -> (x <= y?=w320:bool)
        n207 = And(x=w320, y=w315) -> (x .and. y?=w311:bool)
        n208 = Greater Or Equal?(x=w308, y=180) -> (x >= y?=w309:bool)
        n209 = case shown="假" w311 {
          tunnel: w310 -> [w326 w336]
          tunnel: w309 -> [w327 _]
          tunnel: w308 -> [w325 _]
          tunnel: [w324 _] -> w307
          frame False {
            n210 = case shown="真" w327 {
              tunnel: w326 -> [_ w333]
              tunnel: w325 -> [w328 _]
              tunnel: [w328 _] -> w324
              frame False {
              }
              frame True {
                n211 = Enqueue Element(queue=w333, element=校准步骤."待机" ("元素")) -> ()  [unwired: 2 in, 3 out]
                n212 = global read "多参数全局变量.vi" "多参数编号"() -> (w329:string)
                n213 = Concatenate Strings(w329, "校准超时，校准将停止！" ("消息")) -> (w330:string)
                n214 = One Button Dialog(message=w330) -> ()  [unwired: 1 in, 1 out]
              }
            }
          }
          frame True {
            n215 = Enqueue Element(queue=w336, element=校准步骤."第三点校准写入" ("元素"), timeout in ms (-1)=1000 ("超时毫秒(-1)")) -> ()  [unwired: 1 in, 3 out]
          }
        }
        n216 = Format Into String(format string="正在进行第三点校准,校准可能需要几分钟,请耐性等待,已进行%d秒." ("格式字符串"), w307) -> (resulting string=w322:string)  [unwired: 2 in, 1 out]
      }
      frame "第三点校准写入" {
        n217 = Increment(x=w340) -> (x+1=w339:i32)
        n218 = case shown="2" w339 {
          tunnel: w338 -> [_ _ w349]
          frame 0, Default {
          }
          frame 1 {
            n219 = local read "当前信号值"() -> (→"第三点校准值":dbl)
          }
          frame 2 {
            n220 = local read "三点标液3"() -> (w344:u16)
            n221 = case shown="7" w344 {
              tunnel: [u16 49 ("数值") u16 50 ("数值") u16 51 ("数值") u16 52 ("数值") u16 53 ("数值") u16 54 ("数值") u16 55 ("数值") u16 56 ("数值")] -> w343
              frame 0, Default {
              }
              frame 1 {
              }
              frame 2 {
              }
              frame 3 {
              }
              frame 4 {
              }
              frame 5 {
              }
              frame 6 {
              }
              frame 7 {
              }
            }
            n222 = global read "多参数全局变量.vi" "MB_Serial session"() -> (w346:refnum<class "MB_Master_Serial.lvclass">)
            n223 = call "0035H_pH_第三点校正指令写入.vi"("数值"=w343, "MB_Serial session in"=w346) -> ("error out"=w345:errorcluster)  [unwired: 8 in, 1 out]
            n224 = case shown="错误" w345 {
              tunnel: [校准步骤."校准结果写入" ("元素") 校准步骤."待机" ("元素")] -> w347
              frame No Error {
              }
              frame Error {
                n225 = global read "多参数全局变量.vi" "多参数编号"() -> (w359:string)
                n226 = Concatenate Strings(w359, "校准超时，校准将停止！" ("消息")) -> (w360:string)
                n227 = One Button Dialog(message=w360) -> ()  [unwired: 1 in, 1 out]
              }
            }
            n228 = Enqueue Element(queue=w349, element=w347, timeout in ms (-1)=1000 ("超时毫秒(-1)")) -> ()  [unwired: 1 in, 3 out]
          }
        }
      }
      frame "第三点校准失败" {
      }
      frame "校准结果写入" {
        n229 = local read "校准模式"() -> (w367:enum16{"两点校准", "单点校准", "三点校准"})
        n230 = case shown="\"两点校准\", 默认" w367 {
          tunnel: [w372 w396] -> w364
          frame "两点校准", Default {
            n231 = global read "国弘过程全局变量.vi" "pH"() -> (w371:T3)
            n232 = Unbundle By Name(w371) -> ("电极状态标志"=w370:u16)
            n233 = case shown="2" w370 {
              selector: w370 -> [w374 _ w383 _]
              tunnel: [w373 w378 w382 w387] -> w372
              frame 0, Default {
                n234 = case shown="2" w374 {
                  tunnel: ["校正未正常启动，请重新校正" "第一点校准通过" "第二点校准通过"] -> w373
                  frame 0, Default {
                  }
                  frame 1 {
                  }
                  frame 2 {
                  }
                }
              }
              frame 2 {
                n235 = local read "第一点校准值"() -> (w380:dbl)
                n236 = local read "第二点校准值"() -> (w381:dbl)
                n237 = Format Into String(format string="两点校准结果：第一点校准值：%f；第二点校准值：%f。" ("提示"), w380, w381) -> (resulting string=w378:string)  [unwired: 2 in, 1 out]
              }
              frame 3, 4 {
                n238 = case shown="3, 默认" w383 {
                  tunnel: ["校正失败，电极零点超出范围" "校正失败，电极斜率超出范围"] -> w382
                  frame 3, Default {
                  }
                  frame 4 {
                  }
                }
              }
              frame 5 {
                n239 = local read "第一点校准值"() -> (w389:dbl)
                n240 = local read "第二点校准值"() -> (w390:dbl)
                n241 = local read "第三点校准值"() -> (w386:dbl)
                n242 = Format Into String(format string="三点校准结果：第一点校准值：%f；第二点校准值：%f；第二点校准值：%f。" ("提示"), w389, w390, w386) -> (resulting string=w387:string)  [unwired: 2 in, 1 out]
              }
            }
          }
          frame "单点校准" {
            n243 = local read "当前检测值"() -> (w395:dbl)
            n244 = global read "多参数全局变量.vi" "MB_Serial session"() -> (w393:refnum<class "MB_Master_Serial.lvclass">)
            n245 = local read "标液1"() -> (w394:dbl)
            n246 = Subtract(x=w394, y=w395) -> (x-y=w391:dbl)
            n247 = call "000CH_pH_pH偏移修正值写入.vi"("数值"=w391, "MB_Serial session in"=w393) -> ("error out"=w392:errorcluster)  [unwired: 8 in, 1 out]
            n248 = case shown="无错误" w392 {
              tunnel: [w397 "校准失败"] -> w396
              frame No Error {
                n249 = local read "第一点校准值"() -> (w399:dbl)
                n250 = Format Into String(format string="单点校准结果：\n校准值：%f" ("提示"), w399) -> (resulting string=w397:string)  [unwired: 2 in, 1 out]
              }
              frame Error {
                n251 = One Button Dialog(message="校准失败，请重新校准！" ("消息")) -> ()  [unwired: 1 in, 1 out]
              }
            }
          }
        }
        n252 = Enqueue Element(queue=w369, element=校准步骤."校准结束" ("元素")) -> ()  [unwired: 2 in, 3 out]
        n253 = global read "多参数全局变量.vi" "多参数编号"() -> (w366:string)
        n254 = Concatenate Strings(w366, w364) -> (w363:string)
        n255 = One Button Dialog(message=w363) -> ()  [unwired: 1 in, 1 out]
        n256 = call "操作日志.vi"("日志信息"=w363) -> ("error out"=w365:errorcluster)  [unwired: 10 in]
      }
      frame "校准结束" {
        n257 = local read "提示"() -> (w402:string)
      }
    }
    "提示" <- w120
  }
